vi "bujujiao.vi"(10 "stepnum":u16=2 max=32767, 11 "OK Button":bool) -> ()   [LabVIEW 2015]
uses:
  <vilib>/Instr/_visa.llb/VISA Configure Serial Port (Instr).vi
panel:
  in  "error in (no error)":errorcluster
  out "error out":errorcluster
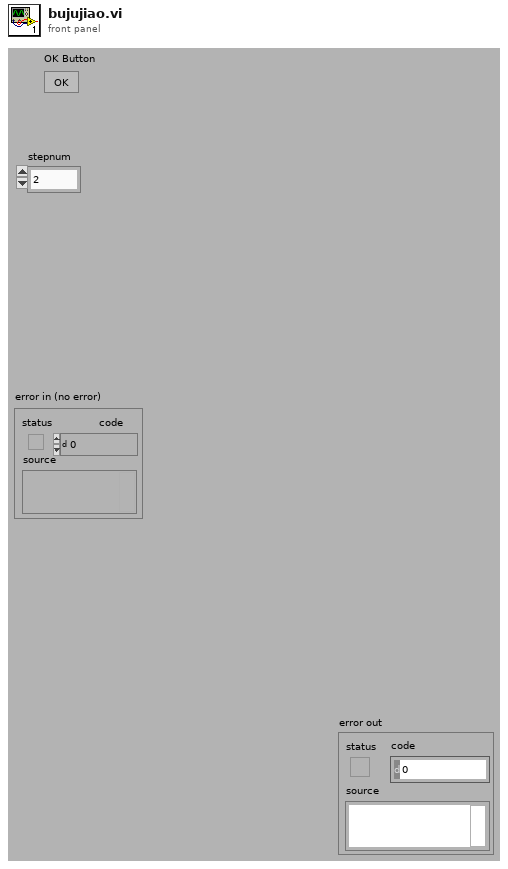
[diagram p1: front panel]
types:
  T1 = enum16{"big-endian, network order", "native, host order", "little-endian"}
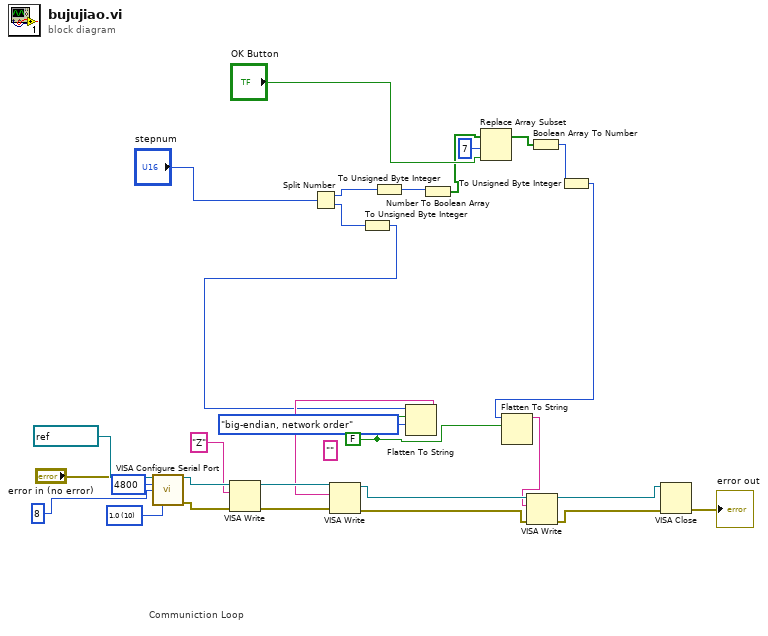
[diagram p0: block diagram]
diagram:
  (unwired) "" ("data string")
  w22 = u16 10 items=["1.0"=10, "1.5"=15, "2.0"=20] ("stop bits (10: 1 bit)")
  w16 = FALSE ("prepend array or string size? (T)")
  # "Communiction Loop"
  n1 = call-poly "VISA Configure Serial Port"("VISA resource name"=refnum<visa-resource-name> "COM1", "baud rate (9600)"=u32 4800, "data bits (8)"=u16 8, "error in (no error)"="error in (no error)", "stop bits (10: 1 bit)"=w22) -> ("VISA resource name out"=w30:refnum<visa-resource-name>, "error out"=w26:errorcluster)  [unwired: 9 in]
  n2 = VISA Write(VISA resource name=w30, write buffer="Z", error in (no error)=w26) -> (VISA resource name out=w24:refnum<visa-resource-name>, error out=w23:errorcluster)  [unwired: 1 out]
  n3 = Split Number(x="stepnum") -> (hi(x)=w9:u8, lo(x)=w10:u8)
  n4 = To Unsigned Byte Integer(number=w10) -> (unsigned 8bit integer=w2:u8)
  n5 = To Unsigned Byte Integer(number=w9) -> (unsigned 8bit integer=w6:u8)
  n6 = Flatten To String(anything=w2, prepend array or string size? (T)=w16, byte order (0:big-endian, network order)=T1."big-endian, network order") -> (data string=w13:string)  [unwired: 1 in, 2 out]
  n7 = VISA Write(VISA resource name=w24, write buffer=w13, error in (no error)=w23) -> (VISA resource name out=w19:refnum<visa-resource-name>, error out=w17:errorcluster)  [unwired: 1 out]
  n8 = Number To Boolean Array(number=w6) -> (Boolean array=w5:bool[])
  n9 = Replace Array Subset(array=w5, new element="OK Button", index=7) -> (w4:bool[])
  n10 = Boolean Array To Number(Boolean array=w4) -> (number=w3:u32)
  n11 = To Unsigned Byte Integer(number=w3) -> (unsigned 8bit integer=w1:u8)
  n12 = Flatten To String(anything=w1, prepend array or string size? (T)=w16) -> (data string=w18:string)  [unwired: 2 in, 2 out]
  n13 = VISA Write(VISA resource name=w19, write buffer=w18, error in (no error)=w17) -> (VISA resource name out=w15:refnum<visa-resource-name>, error out=w14:errorcluster)  [unwired: 1 out]
  n14 = VISA Close(VISA resource name=w15, error in (no error)=w14) -> (error out=→"error out":errorcluster)
